vi "main.vi"(8 "error in":cluster{"状态":bool, "代码":i32, "源":string}) -> (0 "error out":cluster{"状态":bool, "代码":i32, "源":string} caption="错误输出")   [LabVIEW 2015, in "Debug.lvlib"]
uses:
  Debug.lvlib
  Support/Main State.ctl
panel:
  in  "Filter Noise":bool
  in  "停止按钮":bool
  in  "Py Adjust":bool
  in  "Camera":bool
  in  "Ascan":bool
  # "Engineering"
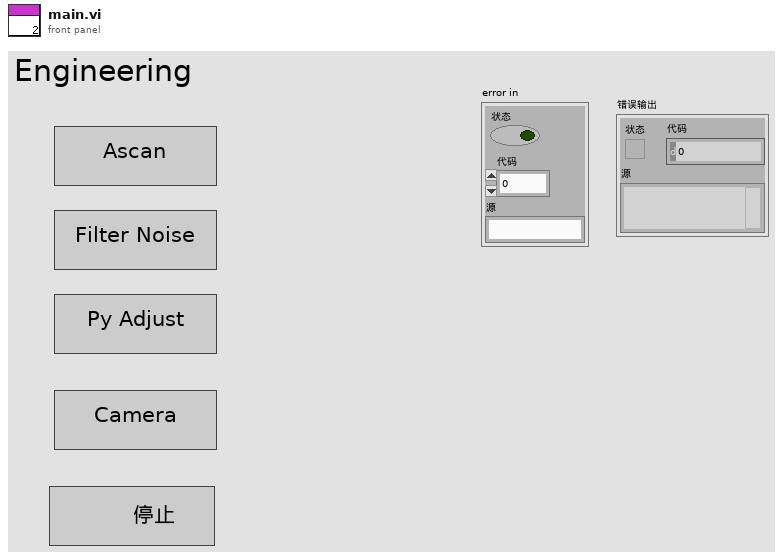
[diagram p1: front panel]
types:
  T1 = typedef "Debug.lvlib/Main State.ctl" = enum16{"Initialize", "Ascan", "Filter Noise", "Py Adjust", "Camera", "Wait For Event", "Exit"}
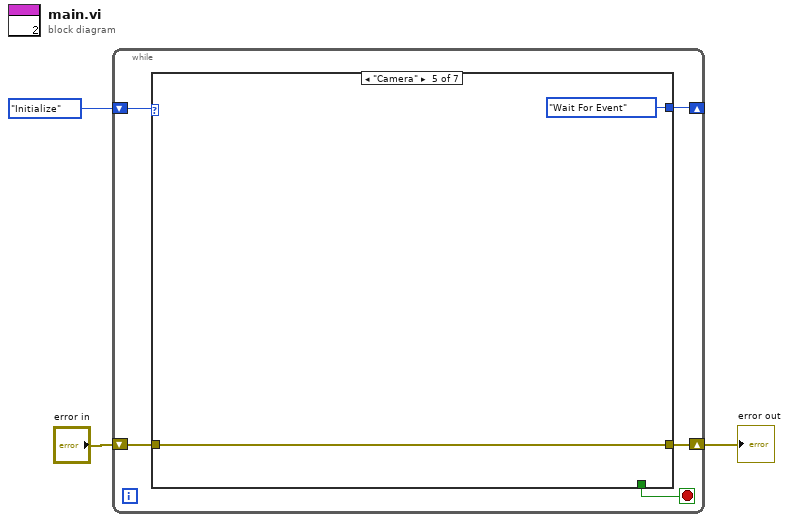
[diagram p0: block diagram]
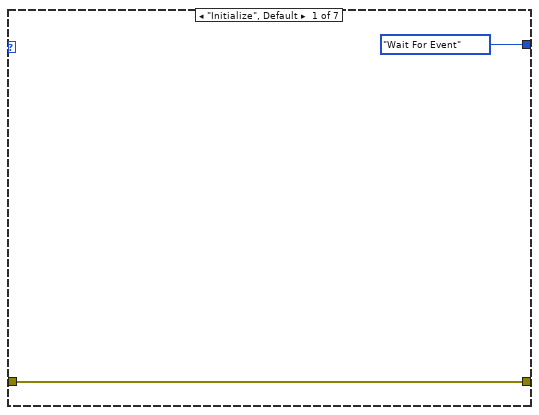
[diagram p2: hidden frame]
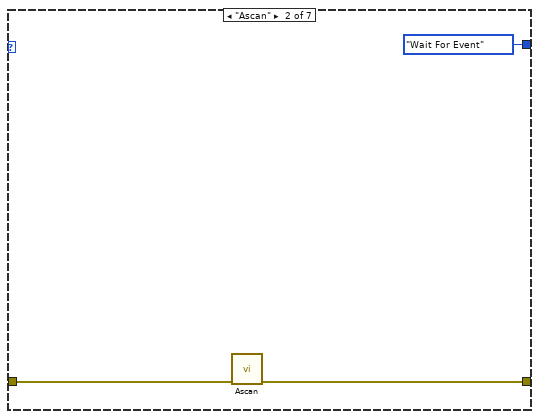
[diagram p3: hidden frame]
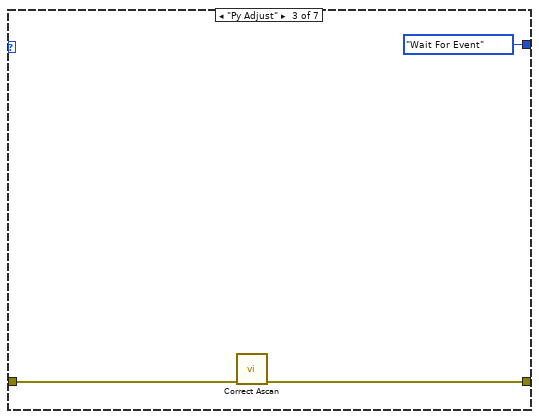
[diagram p4: hidden frame]
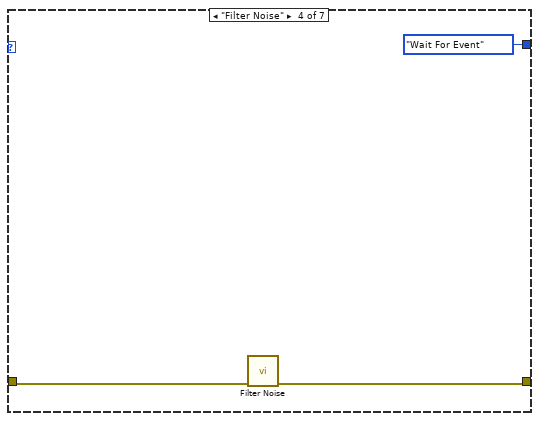
[diagram p5: hidden frame]
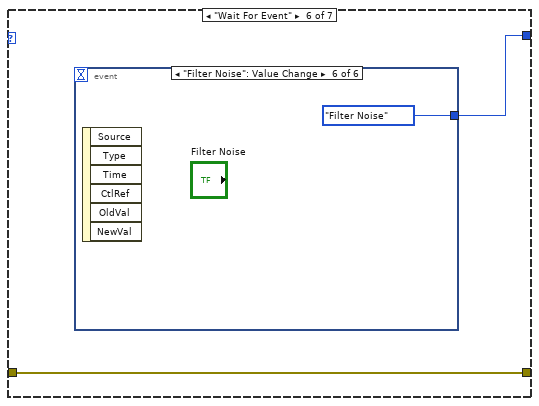
[diagram p6: hidden frame]
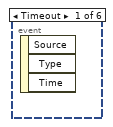
[diagram p7: hidden frame]
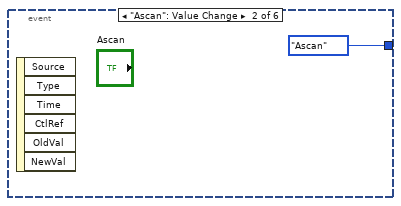
[diagram p8: hidden frame]
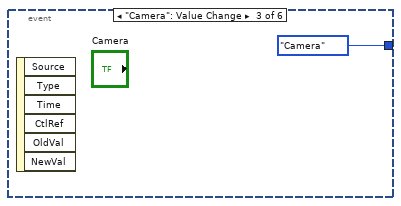
[diagram p9: hidden frame]
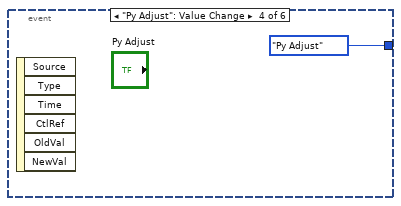
[diagram p10: hidden frame]
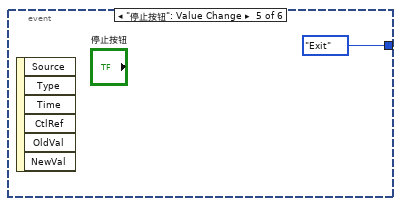
[diagram p11: hidden frame]
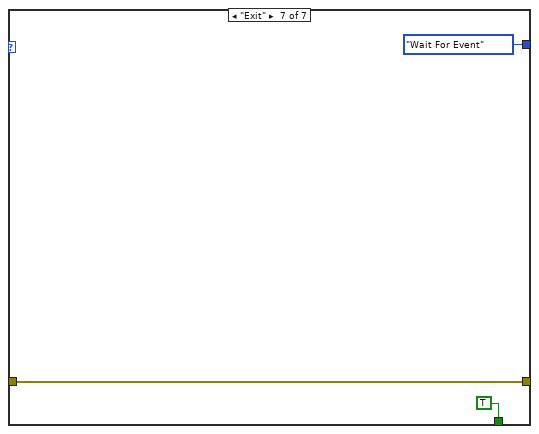
[diagram p12: hidden frame]
diagram:
  n1 = while {
    shift-right: [w7] -> _
    shift-left: Main_State."Initialize" ("Calculation Distance State") -> [w8]
    shift-right: [w6] -> w1
    shift-left: "error in" -> [w5]
    stop <- w4 stop-if-true
    n2 = case shown="\"Camera\"" w8 {
      tunnel: [Main_State."Wait For Event" ("Calculation Distance State") Main_State."Wait For Event" ("Calculation Distance State") Main_State."Wait For Event" ("Calculation Distance State") Main_State."Wait For Event" ("Calculation Distance State") Main_State."Wait For Event" ("Calculation Distance State") w23 Main_State."Wait For Event" ("Calculation Distance State")] -> w7
      tunnel: [w9 w12 w14 w17 w20 w22 w29] -> w6
      tunnel: w5 -> [w9 w11 w15 w18 w20 w22 w29]
      tunnel: [_ _ _ _ _ _ TRUE] -> w4
      frame "Initialize", Default {
      }
      frame "Ascan" {
        n3 = call "Ascan.vi"("error in (no error)"=w11) -> ("error out"=w12:cluster{"状态":bool, "代码":i32, "源":string})  [unwired: 10 in]
      }
      frame "Py Adjust" {
        n4 = call "Correct Ascan.vi"("error in"=w15) -> ("error out"=w14:errorcluster)  [unwired: 10 in]
      }
      frame "Filter Noise" {
        n5 = call "Filter Noise.vi"("error in"=w18) -> ("error out"=w17:errorcluster)  [unwired: 10 in]
      }
      frame "Camera" {
      }
      frame "Wait For Event" {
        n6 = event shown="[5] \"Filter Noise\": Value Change" {
          selector: _ -> [_ _ _ _ _ _]
          dyn-events: _ -> [_ _ _ _ _ _]
          timeout: _ -> [_ _ _ _ _ _]
          tunnel: [_ Main_State."Ascan" ("Calculation Distance State") Main_State."Camera" ("Calculation Distance State") Main_State."Py Adjust" ("Calculation Distance State") Main_State."Exit" ("Calculation Distance State") Main_State."Filter Noise" ("Calculation Distance State")] -> w23
          event Timeout {
            n7 = event-data() -> ()  [unwired: 1 in, 3 out]
          }
          event "Ascan": Value Change {
            n8 = event-data() -> ()  [unwired: 1 in, 6 out]
          }
          event "Camera": Value Change {
            n9 = event-data() -> ()  [unwired: 1 in, 6 out]
          }
          event "Py Adjust": Value Change {
            n10 = event-data() -> ()  [unwired: 1 in, 6 out]
          }
          event "停止按钮": Value Change {
            n11 = event-data() -> ()  [unwired: 1 in, 6 out]
          }
          event "Filter Noise": Value Change {
            n12 = event-data() -> ()  [unwired: 1 in, 6 out]
          }
        }
      }
      frame "Exit" {
      }
    }
  }
  "error out" <- w1
